vi "Команда обмена 71 (ручное упр. ВНИЗ) (SubVI).vi"(1 "Шаг перехода":string, 7 "error in":errorcluster, 9 "TCP connection ID":refnum<k5>) -> (27 "error out":errorcluster)   [LabVIEW 2013]
doc: "Команда 71 - принудительный переход вниз"
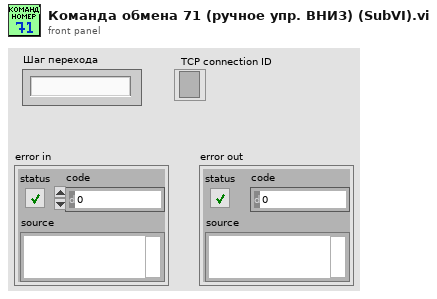
[diagram p1: front panel]
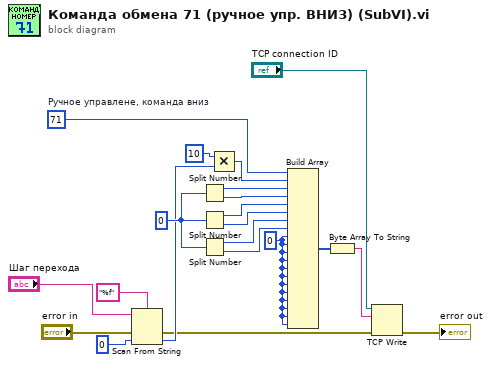
[diagram p0: block diagram]
diagram:
  w9 = u16 0 ("element")
  w21 = u16 0 ("element")
  w11 = u8 71  # Ручное управлене, команда вниз
  n1 = Scan From String(format string="%f", input string="Шаг перехода", error in="error in", default 1=u8 0 ("element")) -> (error out=w1:errorcluster, output 1=w4:u8)  [unwired: 1 in, 2 out]
  n2 = Split Number(x=w9) -> (hi(x)=w15:u8, lo(x)=w16:u8)
  n3 = Split Number(x=w9) -> (hi(x)=w19:u8, lo(x)=w20:u8)
  n4 = Split Number(x=w9) -> (hi(x)=w17:u8, lo(x)=w18:u8)
  n5 = Multiply(x=u8 10 ("element"), y=w4) -> (x*y=w3:u8)
  n6 = Build Array(w11, w3, w15, w16, w19, w20, w17, w18, w21, w21, w21, w21, w21, w21, w21, w21, w21, w21, w21, w21) -> (w12:u16[])
  n7 = Byte Array To String(unsigned byte array=w12) -> (string=w13:string)
  n8 = TCP Write(connection ID="TCP connection ID", data in=w13, error in (no error)=w1) -> (error out=→"error out":errorcluster)  [unwired: 1 in, 2 out]
